vi "Read AppOutput.vi"(8 "error in (no error)":errorcluster, 11 "VisualizeAppRingdown in":refnum<class "VisualizeAppRingdown.lvclass">) -> (0 "error out":errorcluster, 2 "RingdownOutput":T1, 3 "VisualizeAppRingdown out":refnum<class "VisualizeAppRingdown.lvclass">)   [LabVIEW 2014, in "Visualization.lvlib" / "VisualizeAppRingdown.lvclass"]
uses:
  VisualizeAppRingdown.lvclass
  Modules/AppPlugins/RingdownPlugin/PublicAPI/TypeDef/RingdownOutput.ctl
  VisualizeAppRingdown.lvclass/VisualizeAppRingdown.ctl
  Modules/AppPlugins/RingdownPlugin/RingdownPlugin.lvclass
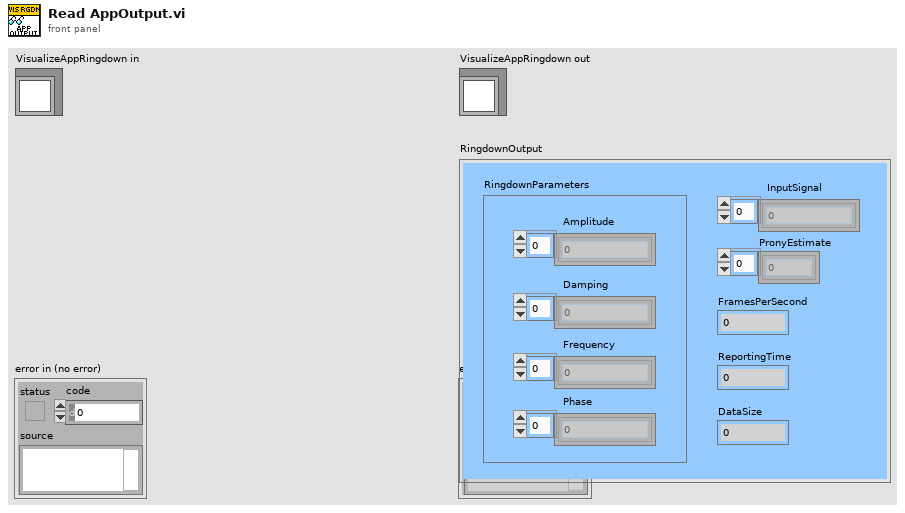
[diagram p1: front panel]
types:
  T1 = typedef "AppPlugins.lvlib/RingdownPlugin.lvclass/RingdownOutput.ctl" = cluster{"FramesPerSecond":dbl, "PronyEstimate":dbl[], "RingdownParameters":cluster{"Amplitude":dbl[], "Damping":dbl[], "Frequency":dbl[], "Phase":dbl[]}, "ReportingTime":dbl, "DataSize":u32, "InputSignal":dbl[]}
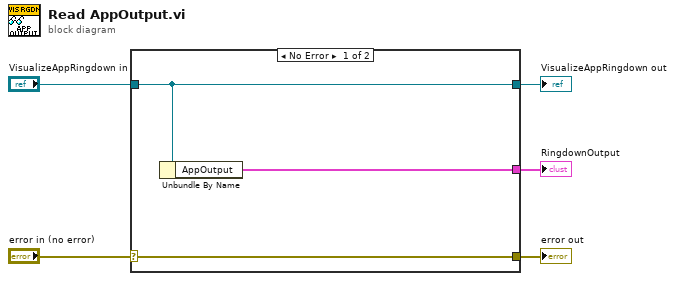
[diagram p0: block diagram]
diagram:
  n1 = case shown="No Error" "error in (no error)" {
    selector: "error in (no error)" -> [w8 w9]
    tunnel: [w8 w9] -> w4
    tunnel: [w7 w10] -> w2
    tunnel: "VisualizeAppRingdown in" -> [w7 w10]
    tunnel: [w6 _] -> w1
    frame No Error {
      n2 = Unbundle By Name(w7) -> ("AppOutput"=w6:T1)
    }
    frame Error {
    }
  }
  "error out" <- w4
  "VisualizeAppRingdown out" <- w2
  "RingdownOutput" <- w1
